vi "Read Image File_example.vi"() -> ()   [LabVIEW 2020]
doc: "This example shows how to open, read, and display images in NI Vision. The image control is in Snapshot mode so when you dispose the image, the control image stays in memory."
uses:
  <vilib>/vision/NI_Vision_Development_Module.lvlib
panel:
  out "XY Graph":cluster{"X":dbl, "Y":dbl}[](graph)
  out "Points":i32[][](array[numeric])
  out "Array 2":u32[](array[numeric])
  out "Array":u32[](array[numeric])
  out "Contours":T1(array[cluster])
  out "Global Rectangle":i32[](array[numeric])
  out "ROI":T2
  out "Core Image":T3(plugin-control)
  out "error out":errorcluster
  out "Threshold":T3(plugin-control) caption="Threshold Image"
  out "Image Pixels (I16) 2":i16[][](array[numeric])
  out "Image Pixels (I16)":i16[][](array[numeric])
  out "CropedImage":T3(plugin-control)
  in  "Optional Rectangle":i32[](array[numeric])
  in  "Left image intensity":cluster{i16, i16}(slide)={0, 2048} scale=0.0..4095.0
  in  "stop":bool
  out "Intensity Graph":i16[][](graph)
  in  "Path":path
  out "Image":T3(plugin-control)
  # "Overview: Demonstrate the use of the AVI functions to read an AVI movie file.\nRequirements: Vision Development Software.\nInstructions: Run the VI."
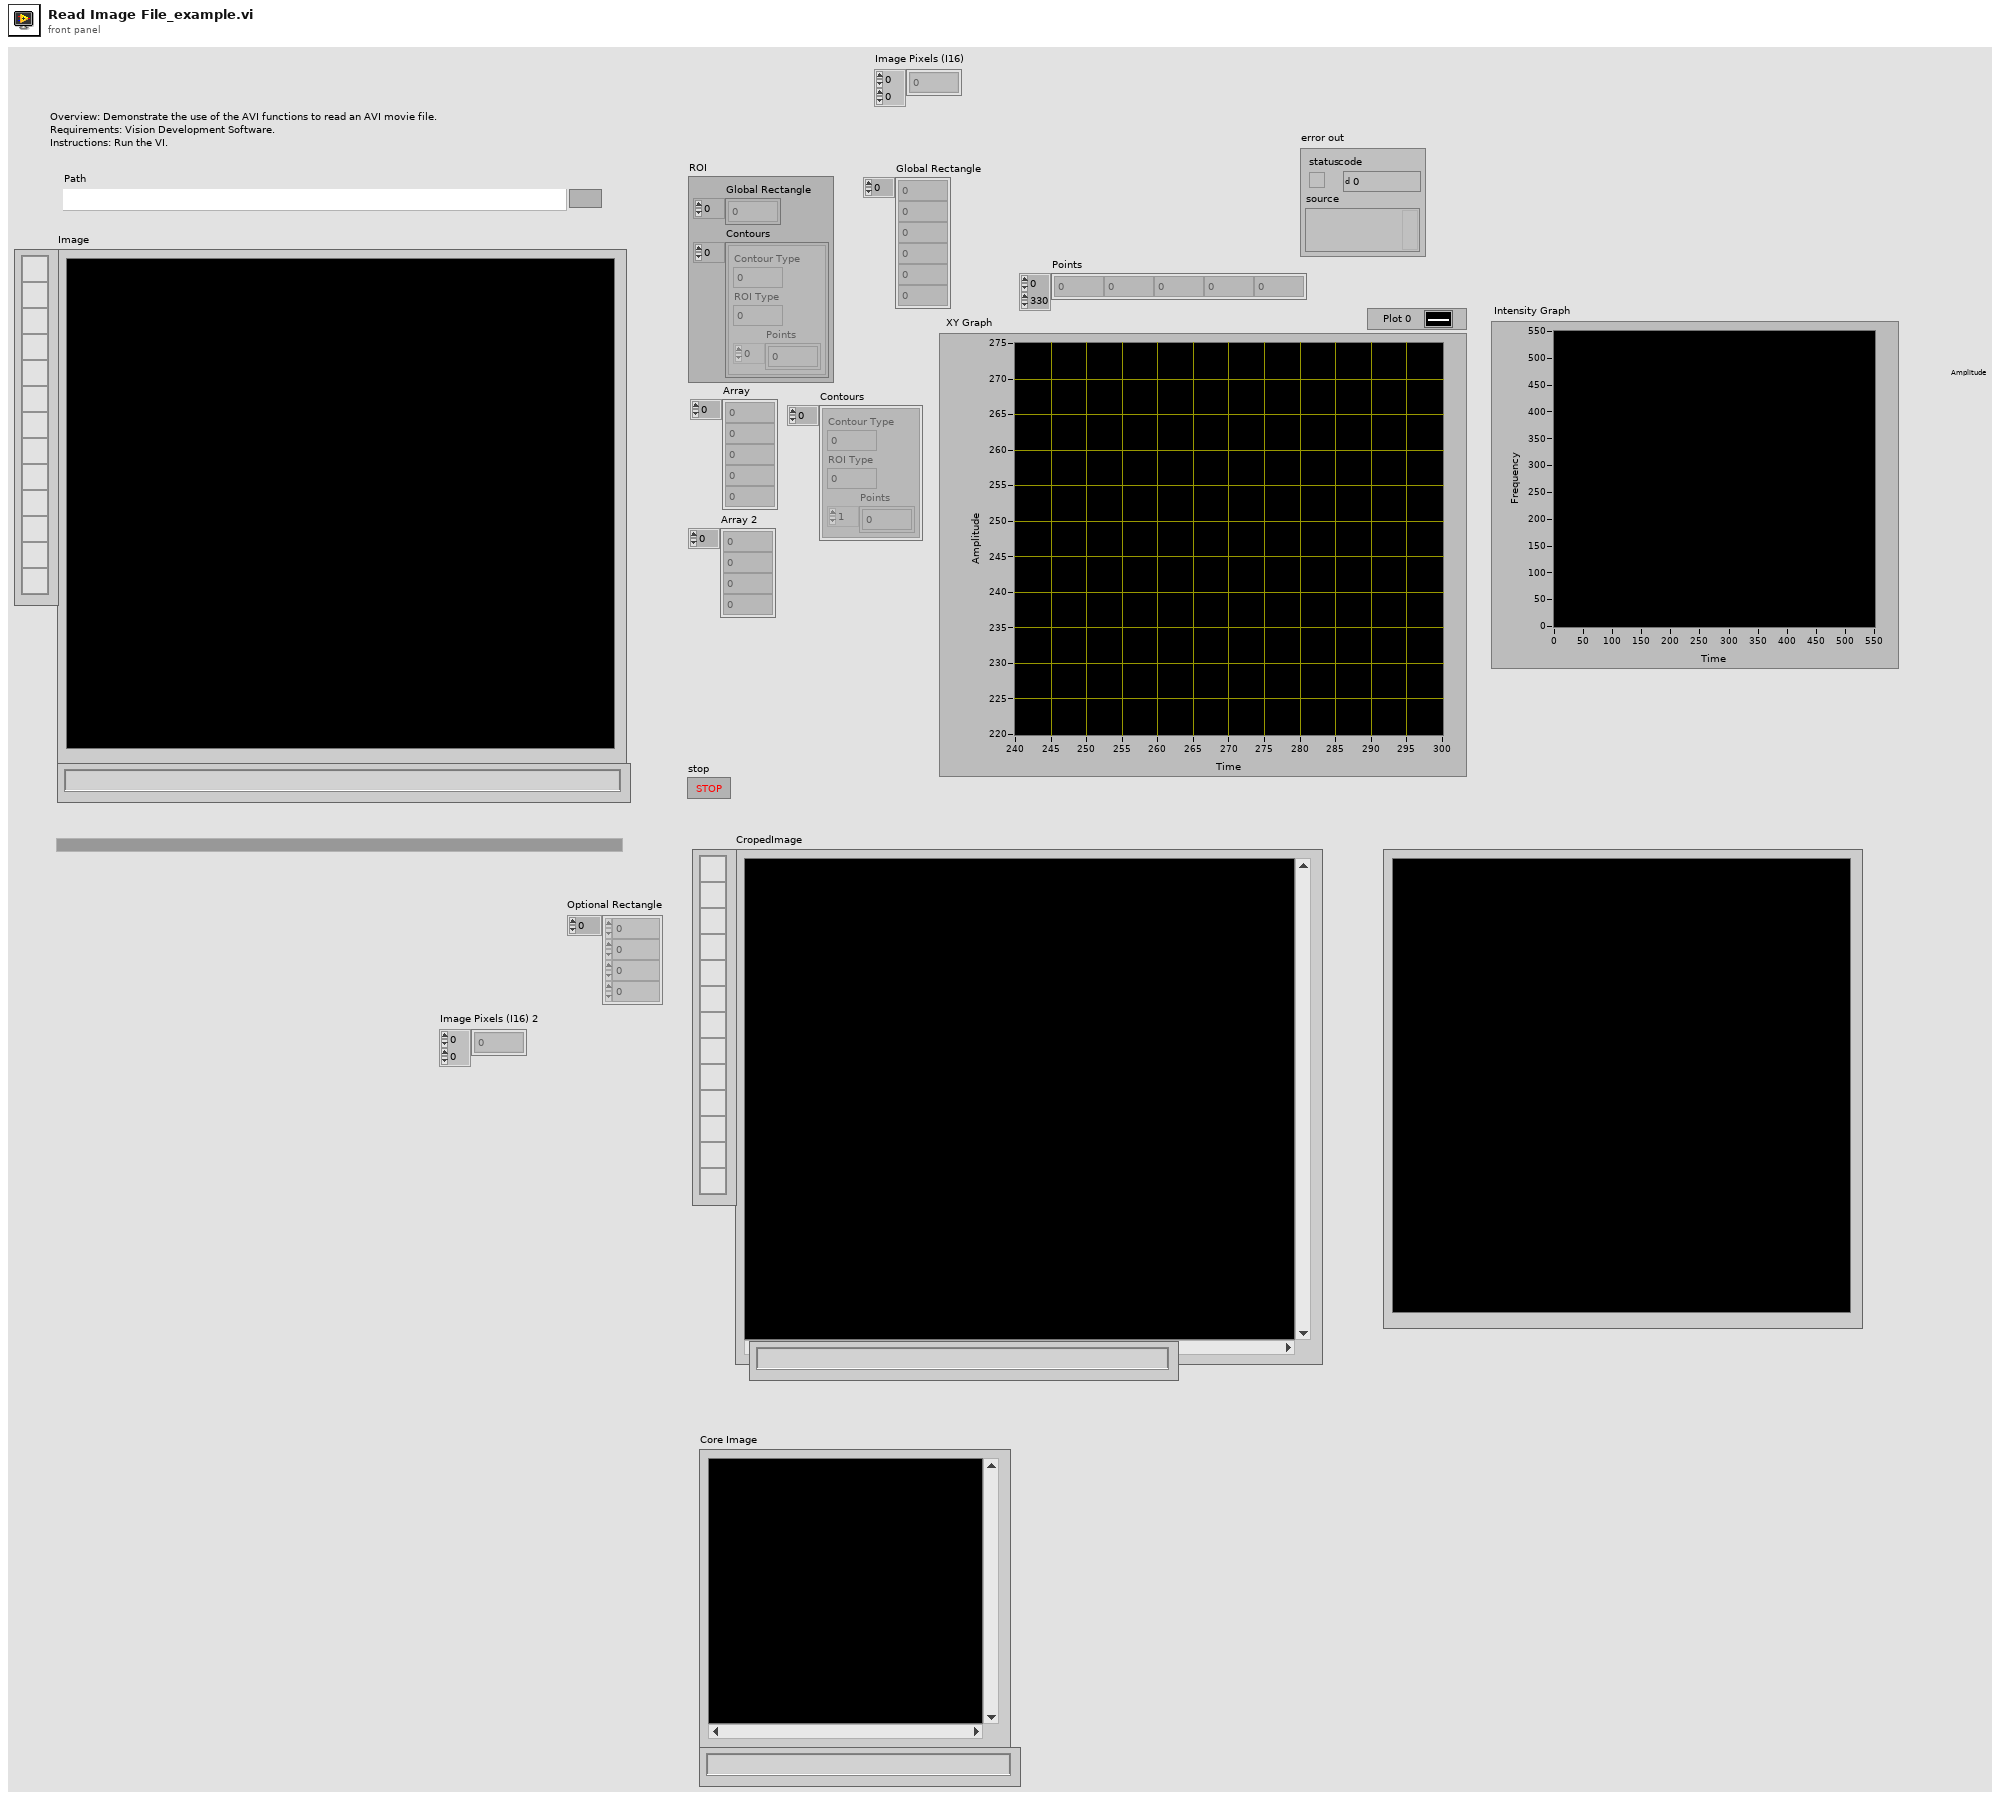
[diagram p1: front panel]
types:
  T1 = cluster{"Contour Type":u32, "ROI Type":u32, "Points":i32[]}[]
  T2 = cluster{"Global Rectangle":i32[], "Contours":cluster{"Contour Type":u32, "ROI Type":u32, "Points":i32[]}[]}
  T3 = typedef "IMAQ Image.ctl" = refnum<image>
  T4 = cluster{"Conversion Method":u32, "Minimum Value":i32, "Maximum Value":i32, "Number Of Shifts":i32}
  T5 = typedef "Image Type" = u32
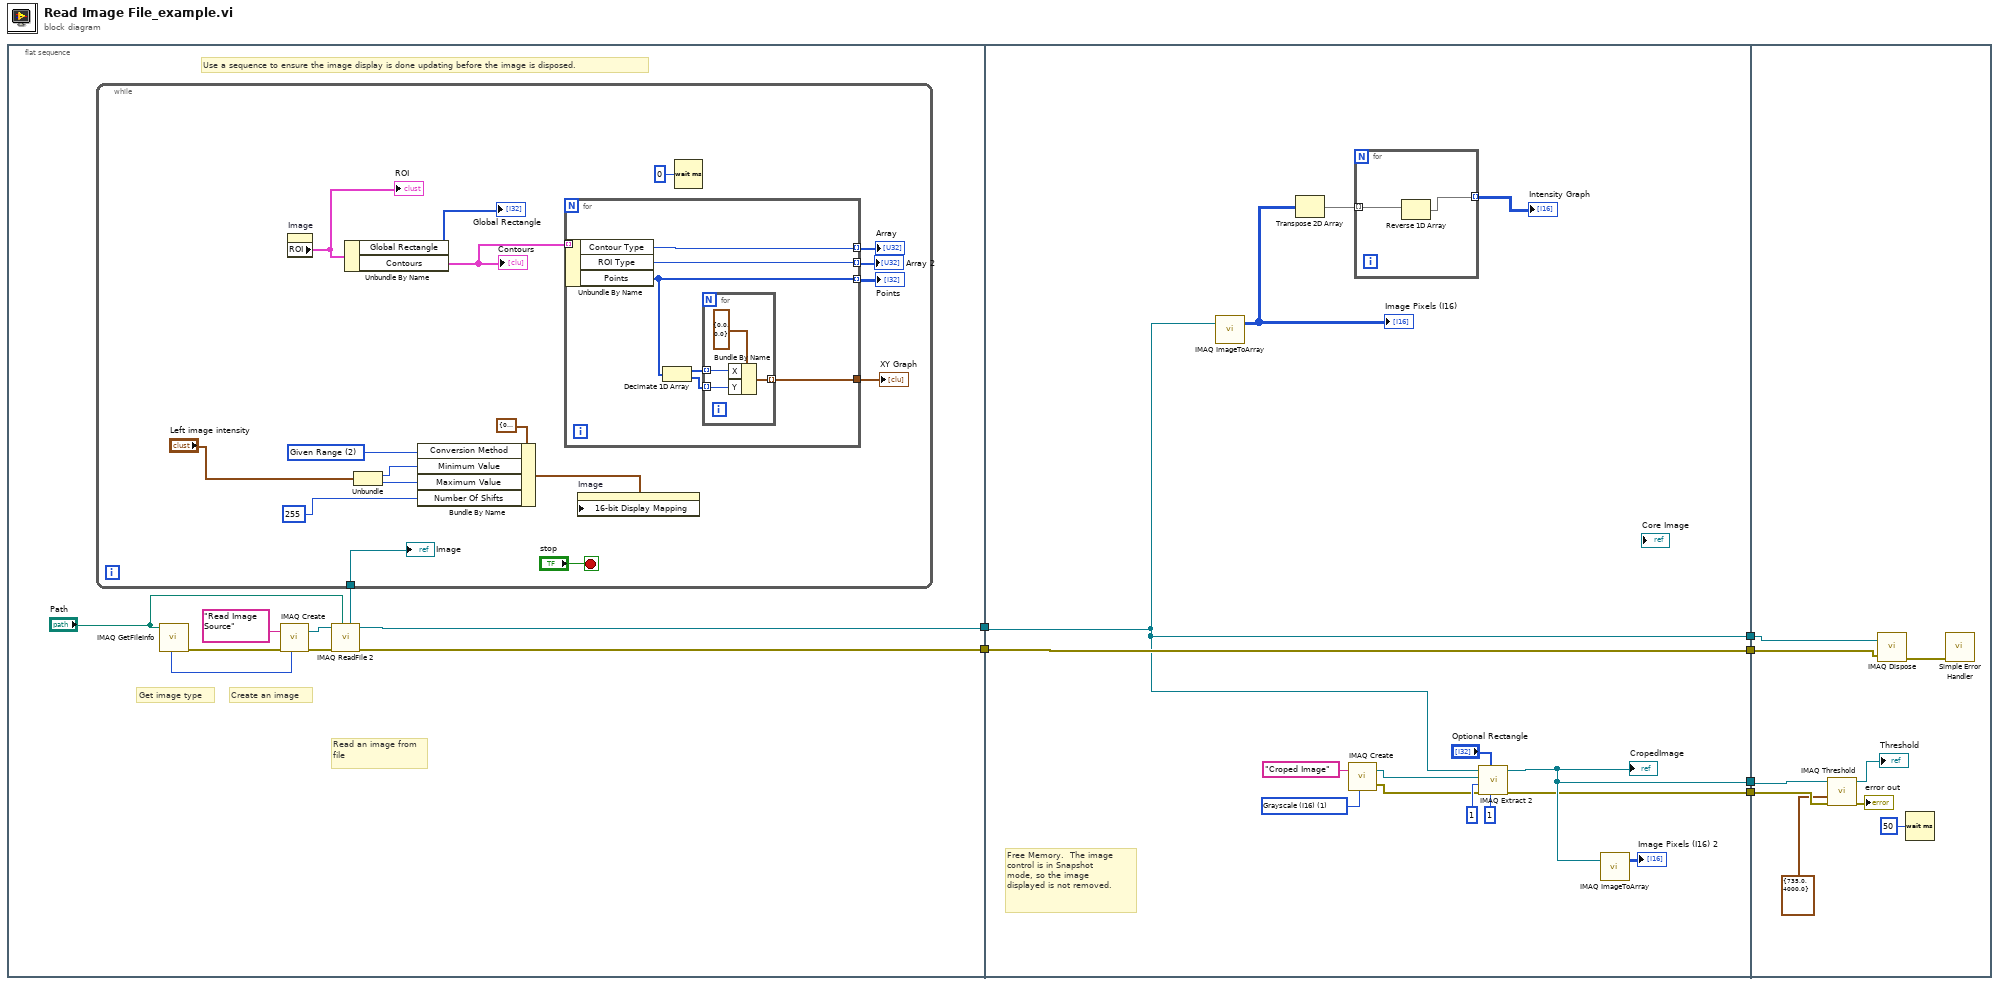
[diagram p0: block diagram]
diagram:
  n1 = flat-sequence {
    tunnel: [w8] -> w6
    tunnel: [w7] -> w5
    tunnel: w6 -> [w49]
    tunnel: w5 -> [w50]
    tunnel: [w50] -> w4
    tunnel: [w49] -> w3
    tunnel: [w44] -> w2
    tunnel: [w43] -> w1
    tunnel: w4 -> [w68]
    tunnel: w3 -> [w67]
    tunnel: w2 -> [w65]
    tunnel: w1 -> [w64]
    frame #0 {
      # "Use a sequence to ensure the image display is done updating before the image is disposed."
      # "Get image type"
      # "Read an image from file"
      # "Create an image"
      n2 = call "IMAQ GetFileInfo"("File Path"="Path") -> ("error out"=w11:errorcluster, "Image Type"=w12:T5)  [unwired: 4 in, 5 out]
      n3 = call "IMAQ Create"("Image Name"="Read Image Source", "Image Type"=w12, "error in (no error)"=w11) -> ("New Image"=w13:T3, "error out"=w14:errorcluster)  [unwired: 2 in]
      n4 = call "IMAQ ReadFile 2"("File Path"="Path", "error in (no error)"=w14, "Image"=w13) -> ("error out"=w7:errorcluster, "Image Out"=w8:T3)  [unwired: 4 in, 3 out]
      n5 = while {
        tunnel: w8 -> [w31]
        stop <- "stop" stop-if-true
        w26 = u32 2 items=["Full Dynamic", "Downshift", "Given Range", "90% Dynamic", "Given Percent Range"] ("Conversion Method (Given Range)")
        n6 = property on="Image" class="ImageControl"() -> ("ROI"=w21:T2)  [unwired: 2 in, 2 out]
        "ROI" <- w21
        n7 = Unbundle By Name(w21) -> ("Global Rectangle"=→"Global Rectangle":i32[], "Contours"=w19:T1)
        "Contours" <- w19
        n8 = Unbundle("Left image intensity") -> (w23:i16, w22:i16)
        n9 = Bundle By Name(cluster=T4 {"Conversion Method"=0, "Minimum Value"=0, "Maximum Value"=0, "Number Of Shifts"=0} ("16-bit Display Mapping:All Elements"), "Conversion Method"=w26, "Minimum Value"=w23, "Maximum Value"=w22, "Number Of Shifts"=255 ("Number Of Shifts (255)")) -> (w27:T4)
        n10 = for {
          tunnel: w19 -> [w38] mode=indexing
          tunnel: [w37] -> w18 mode=indexing
          tunnel: [w36] -> w17 mode=indexing
          tunnel: [w35] -> w16 mode=indexing
          tunnel: [w32] -> w15
          n11 = Unbundle By Name(w38) -> ("Contour Type"=w37:u32, "ROI Type"=w36:u32, "Points"=w35:i32[])
          n12 = Decimate 1D Array(w35) -> (w34:i32[], w33:i32[])
          n13 = for {
            tunnel: w34 -> [w41] mode=indexing
            tunnel: w33 -> [w40] mode=indexing
            tunnel: [w39] -> w32 mode=indexing
            n14 = Bundle By Name(cluster=cluster{"X":dbl, "Y":dbl} {"X"=0.0, "Y"=0.0}, "X"=w41, "Y"=w40) -> (w39:cluster{"X":dbl, "Y":dbl})
          }
        }
        "Array" <- w18
        "Array 2" <- w17
        "Points" <- w16
        "XY Graph" <- w15
        n15 = property on="Image" class="ImageControl"("16-bit Display Mapping"=w27) -> ()  [unwired: 2 in, 2 out]
        n16 = Wait (ms)(milliseconds to wait=u32 0) -> ()  [unwired: 1 out]
        "Image" <- w31
      }
    }
    frame #1 {
      w56 = T5 1 items=["Grayscale (U8)", "Grayscale (I16)", "Grayscale (SGL)", "Complex (CSG)", "RGB (U32)", "HSL (U32)", "RGB (U64)", "Grayscale (U16)"] ("Image Type")
      # "Free Memory.  The image control is in Snapshot mode, so the image displayed is not removed."
      n17 = call "IMAQ ImageToArray"("Image"=w49) -> ("Image Pixels (I16)"=w45:i16[][])  [unwired: 3 in, 4 out]
      "Image Pixels (I16)" <- w45
      n18 = Transpose 2D Array(2D array=w45) -> (transposed array=w47:i16[][])
      n19 = call "IMAQ Create"("Image Name"="Croped Image", "Image Type"=w56) -> ("New Image"=w51:T3, "error out"=w52:errorcluster)  [unwired: 3 in]
      n20 = for {
        tunnel: w47 -> [w59] mode=indexing
        tunnel: [w58] -> w46 mode=indexing
        n21 = Reverse 1D Array(array=w59) -> (reversed array=w58:i16[])
      }
      "Intensity Graph" <- w46
      n22 = call "IMAQ Extract 2"("Y Step Size"=1, "Optional Rectangle"="Optional Rectangle", "error in (no error)"=w52, "X Step Size"=1, "Image Dst"=w51, "Image Src"=w49) -> ("error out"=w43:errorcluster, "Image Dst Out"=w44:T3)  [unwired: 4 in]
      "CropedImage" <- w44
      n23 = call "IMAQ ImageToArray"("Image"=w44) -> ("Image Pixels (I16)"=→"Image Pixels (I16) 2":i16[][])  [unwired: 3 in, 4 out]
    }
    frame #2 {
      n24 = call "IMAQ Threshold"("error in (no error)"=w64, "Range"=cluster{"Lower value":sgl, "Upper value":sgl} {"Lower value"=735.0, "Upper value"=4000.0}, "Image Src"=w65) -> ("error out"=→"error out":errorcluster, "Image Dst Out"=→"Threshold":T3)  [unwired: 7 in]
      n25 = call "IMAQ Dispose"("Image"=w67, "error in (no error)"=w68) -> ("error out"=w66:errorcluster)  [unwired: 4 in]
      n26 = Wait (ms)(milliseconds to wait=u32 50) -> ()  [unwired: 1 out]
      n27 = call <vilib>:"Simple Error Handler.vi"("error in (no error)"=w66) -> ()  [unwired: 4 in, 5 out]
    }
  }
